vi "Initialize Debug Attribute.vi"(7 "Attribute.StartupBehavior in":refnum<class "Attribute.Debug.lvclass">, 11 "Behavior (Normal)":T1) -> (3 "Attribute.StartupBehavior":refnum<class "Attribute.Debug.lvclass">)   [LabVIEW 2019, in "SMO Debug.lvlib" / "Attribute.Debug.lvclass"]
uses:
  Attribute.Debug.lvclass
  C:/Program Files (x86)/National Instruments/LabVIEW 2019/vi.lib/JKI/JKI SMO/Support/Attribute/Attribute.lvclass
  DebugBehavior.ctl
  <vilib>/JKI/JKI SMO/Definitions/def.SMO/Scope -- Enum.ctl
  <vilib>/JKI/JKI SMO/Support/Attribute/Attribute.lvclass/Attribute.ctl
  Attribute.Debug.lvclass/Attribute.Debug.ctl
  <vilib>/JKI/JKI SMO/Definitions/def.SMO/def.SMO.lvclass
  <vilib>/JKI/JKI SMO/Support/Attribute/Attribute.lvclass
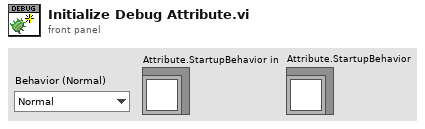
[diagram p1: front panel]
types:
  T1 = typedef "SMO Debug.lvlib/Attribute.Debug.lvclass/DebugBehavior.ctl" = enum16{"Normal", "Debug"}
  T2 = typedef "def.SMO.lvclass/Scope -- Enum.ctl" = enum16{"Public", "Protected", "Private"}
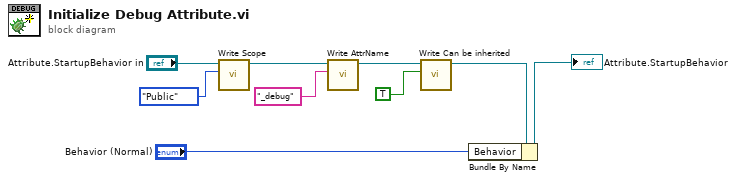
[diagram p0: block diagram]
diagram:
  n1 = call <vilib>:"Write Scope.vi"("Scope"=Scope_--_Enum."Public", "Attribute in"="Attribute.StartupBehavior in") -> ("Attribute out"=w7:refnum<class "Attribute.Debug.lvclass">)  [unwired: 9 in]
  n2 = call <vilib>:"Write AttrName.vi"("Attribute Name"="_debug", "Attribute in"=w7) -> ("Attribute out"=w4:refnum<class "Attribute.Debug.lvclass">)  [unwired: 9 in]
  n3 = call <vilib>:"Write Can be inherited.vi"("Can be inherited"=TRUE, "Attribute in"=w4) -> ("Attribute out"=w3:refnum<class "Attribute.Debug.lvclass">)  [unwired: 8 in, 1 out]
  n4 = Bundle By Name(cluster=w3, "Behavior"="Behavior (Normal)") -> (→"Attribute.StartupBehavior":refnum<class "Attribute.Debug.lvclass">)
